vi "Assignment server.vi"() -> ()   [LabVIEW 2023]
uses:
  Control 1 server.ctl
  <vilib>/Utility/file.llb/Read Delimited Spreadsheet (string).vi
  <vilib>/Utility/file.llb/Write Delimited Spreadsheet (string).vi
  <vilib>/regexp/Match Regular Expression.xnode
panel:
  in  "Tab Control":enum32{"Page 1", "Page 2", "Page 3"}(tab)
  in  "Edit Users":bool
  in  "View Log":bool
  in  "Home Users":bool
  in  "Update users":bool
  in  "Users":string[][](table)
  out "Economy Sales":dbl
  out "Deluxe Sales":dbl
  out "Total Sales":dbl
  in  "Purchase Log":string[][](table)
  in  "Home Purchase":bool
  out "login status":dbl
  out "Logged in?":bool
  out "Password":string
  out "Username":string
  # "ADMIN DASHBOARD"
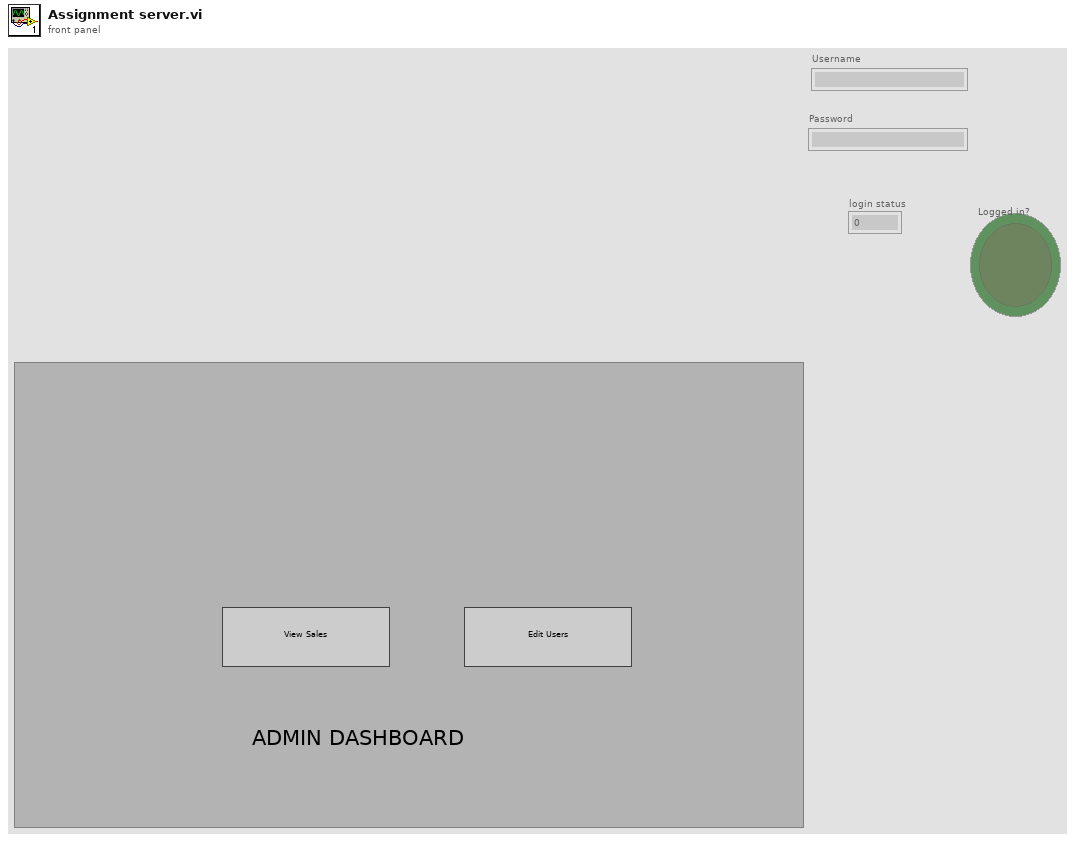
[diagram p1: front panel]
types:
  T1 = typedef "Control 1 server.ctl" = enum16{"init", "login", "logging", "pre-init"}
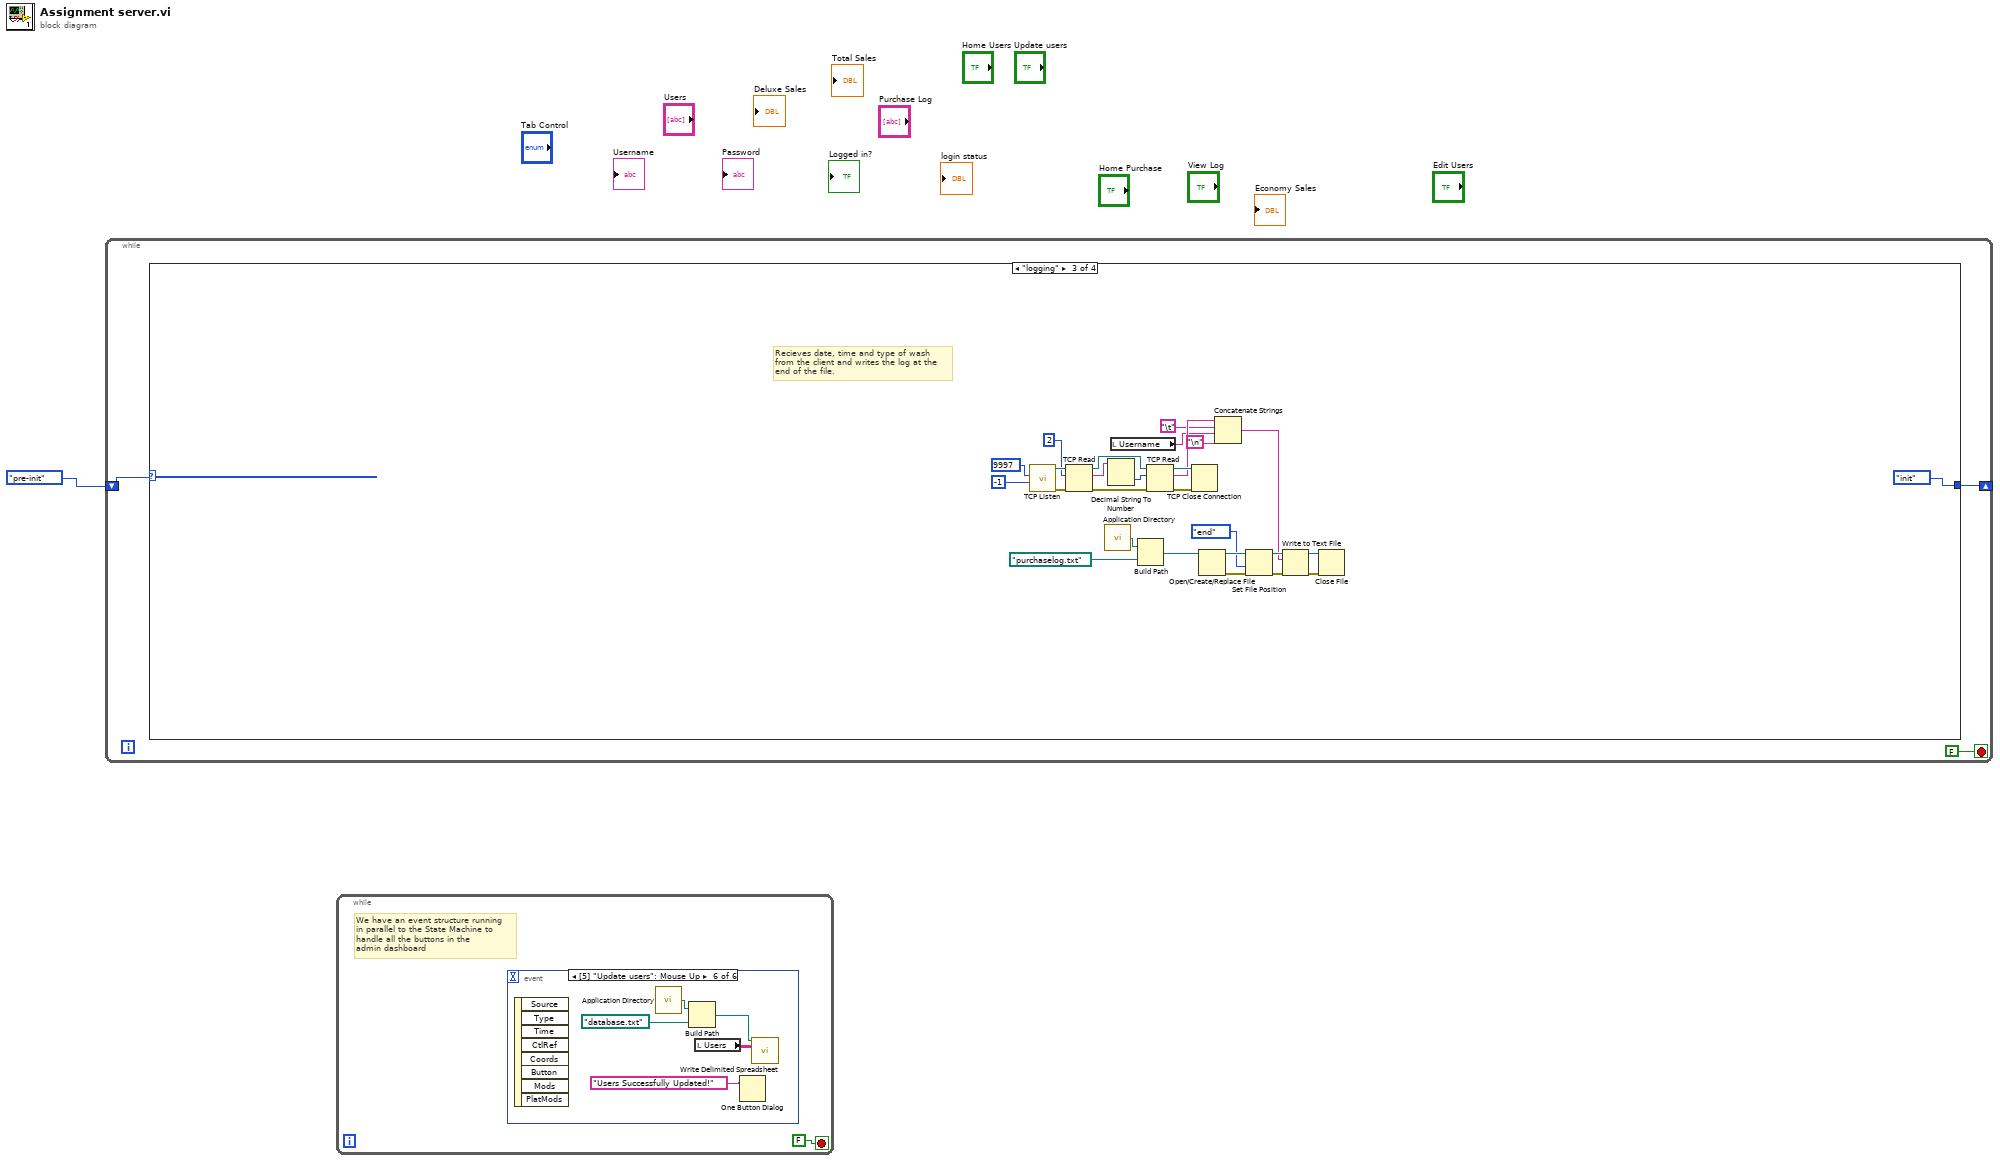
[diagram p0: block diagram]
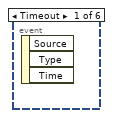
[diagram p2: hidden frame]
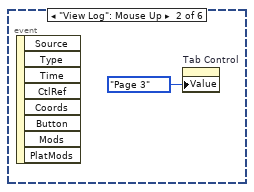
[diagram p3: hidden frame]
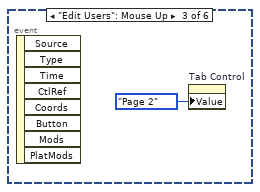
[diagram p4: hidden frame]
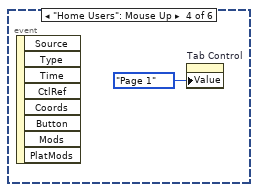
[diagram p5: hidden frame]
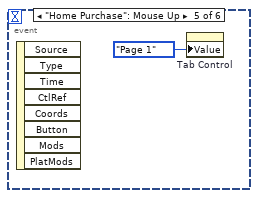
[diagram p6: hidden frame]
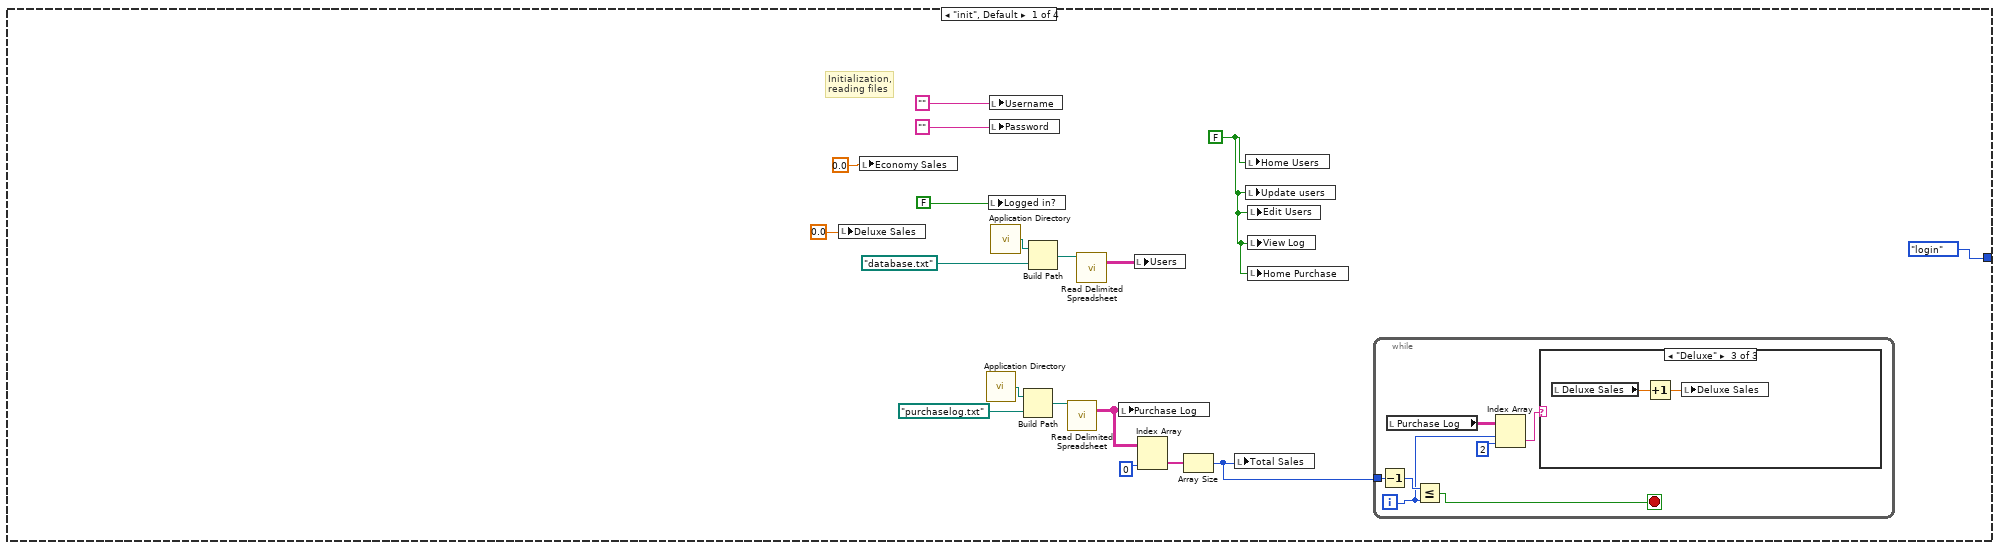
[diagram p7: hidden frame]
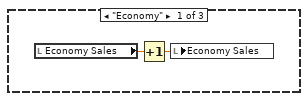
[diagram p8: hidden frame]
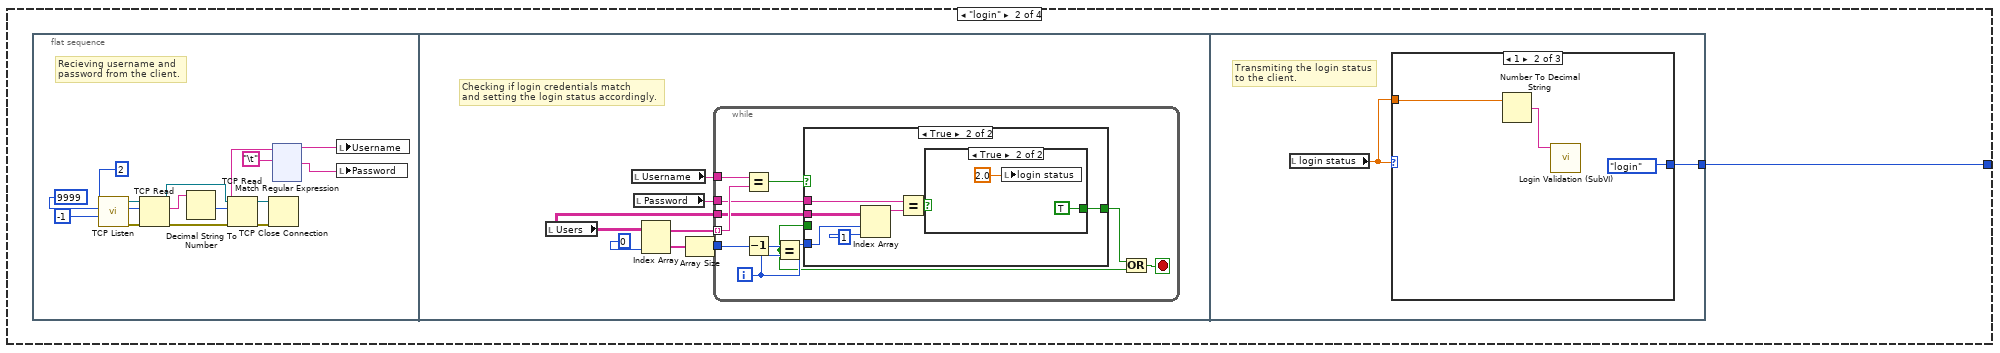
[diagram p10: hidden frame]
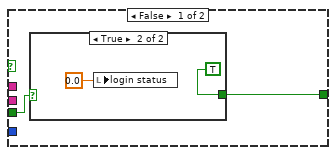
[diagram p11: hidden frame]
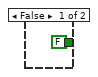
[diagram p12: hidden frame]
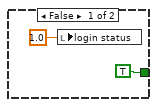
[diagram p13: hidden frame]
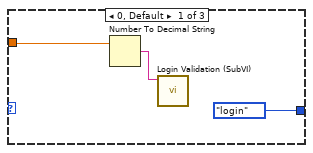
[diagram p14: hidden frame]
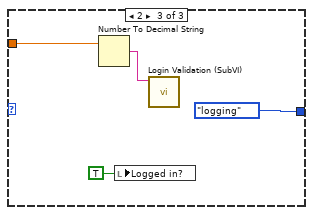
[diagram p15: hidden frame]
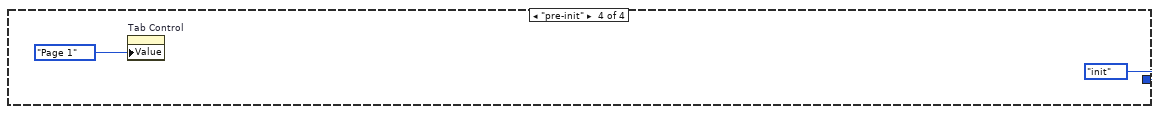
[diagram p16: hidden frame]
diagram:
  n1 = while {
    shift-right: [w2] -> _
    shift-left: Control_1_server."pre-init" -> [w3]
    stop <- FALSE stop-if-true
    n2 = case shown="\"logging\"" w3 {
      tunnel: [Control_1_server."login" w34 Control_1_server."init" Control_1_server."init"] -> w2
      frame "init", Default {
        w12 = FALSE ("Home Users")
        # "Initialization,\nreading files"
        n3 = local write "Deluxe Sales"(0.0 ("Economy Sales:")) -> ()
        n4 = local write "Economy Sales"(0.0 ("Economy Sales:")) -> ()
        n5 = call <vilib>:"Application Directory.vi"() -> ("Application Directory"=w13:path)
        n6 = local write "Logged in?"(FALSE ("Logged in?")) -> ()
        n7 = local write "Username"("" ("Username")) -> ()
        n8 = local write "Password"("" ("Password")) -> ()
        n9 = call <vilib>:"Application Directory.vi"() -> ("Application Directory"=w14:path)
        n10 = Build Path(base path=w13, name or relative path=path "purchaselog.txt") -> (appended path=w15:path)
        n11 = Build Path(base path=w14, name or relative path=path "database.txt") -> (appended path=w17:path)
        n12 = call-poly <vilib>:"Read Delimited Spreadsheet.vi"("file path (dialog if empty)"=w15) -> ("all rows"=w8:string[][])  [unwired: 9 in, 5 out]
        n13 = call-poly <vilib>:"Read Delimited Spreadsheet.vi"("file path (dialog if empty)"=w17) -> ("all rows"=w11:string[][])  [unwired: 9 in, 5 out]
        n14 = local write "Purchase Log"(w8) -> ()
        n15 = local write "Users"(w11) -> ()
        n16 = Index Array(array=w8, index (col)=0) -> (element=w10:string[])  [unwired: 1 in]
        n17 = Array Size(array=w10) -> (size(s)=w7:i32)
        n18 = local write "Total Sales"(w7) -> ()
        n19 = local write "Home Users"(w12) -> ()
        n20 = local write "Update users"(w12) -> ()
        n21 = local write "Edit Users"(w12) -> ()
        n22 = local write "View Log"(w12) -> ()
        n23 = local write "Home Purchase"(w12) -> ()
        n24 = while {
          tunnel: w7 -> [w27]
          i -> [w24]
          stop <- w23 stop-if-true
          n25 = Decrement(x=w27) -> (x-1=w25:i32)
          n26 = local read "Purchase Log"() -> (w29:string[][])
          n27 = Less Or Equal?(x=w25, y=w24) -> (x <= y?=w23:bool)
          n28 = Index Array(array=w29, index (row)=w24, index (col)=2) -> (element=w26:string)
          n29 = case shown="\"Deluxe\"" w26 {
            frame "Economy" {
              n30 = local read "Economy Sales"() -> (w31:dbl)
              n31 = Increment(x=w31) -> (x+1=w30:dbl)
              n32 = local write "Economy Sales"(w30) -> ()
            }
            frame Default {
            }
            frame "Deluxe" {
              n33 = local read "Deluxe Sales"() -> (w33:dbl)
              n34 = Increment(x=w33) -> (x+1=w32:dbl)
              n35 = local write "Deluxe Sales"(w32) -> ()
            }
          }
        }
      }
      frame "login" {
        n36 = flat-sequence {
          tunnel: [w200] -> w34
          frame #0 {
            # "Recieving username and\npassword from the client."
            n37 = call <vilib>:"TCP Listen.vi"("timeout ms (wait forever: -1)"=-1, "port"=u16 9999) -> ("error out"=w48:errorcluster, "connection ID"=w49:refnum<k5>)  [unwired: 5 in, 3 out]
            n38 = TCP Read(connection ID=w49, bytes to read=2, error in (no error)=w48) -> (connection ID out=w36:refnum<k5>, data out=w35:string, error out=w47:errorcluster)  [unwired: 2 in]
            n39 = Decimal String To Number(string=w35) -> (number=w44:i32)  [unwired: 2 in, 1 out]
            n40 = TCP Read(connection ID=w36, bytes to read=w44, error in (no error)=w47) -> (connection ID out=w45:refnum<k5>, data out=w43:string, error out=w46:errorcluster)  [unwired: 2 in]
            n41 = TCP Close Connection(connection ID=w45, error in (no error)=w46) -> ()  [unwired: 1 in, 2 out]
            n42 = xnode ("Match Regular Expression")("input string"=w43, "regular expression"="\t") -> ("before match"=w38:string, "after match"=w37:string)  [unwired: 4 in, 3 out]
            n43 = local write "Username"(w38) -> ()
            n44 = local write "Password"(w37) -> ()
          }
          frame #1 {
            # "Checking if login credentials match\nand setting the login status accordingly."
            n45 = local read "Users"() -> (w170:string[][])
            n46 = local read "Username"() -> (w168:string)
            n47 = local read "Password"() -> (w167:string)
            n48 = Index Array(array=w170, index (col)=0 ("index (row)")) -> (element=w171:string[])  [unwired: 1 in]
            n49 = Array Size(array=w171) -> (size(s)=w172:i32)
            n50 = while {
              tunnel: w172 -> [w183]
              tunnel: w171 -> [w181] mode=indexing
              tunnel: w170 -> [w179]
              tunnel: w168 -> [w174]
              tunnel: w167 -> [w173]
              i -> [w178]
              stop <- w177 stop-if-true
              n51 = Equal?(x=w174, y=w181) -> (x = y?=w180:bool)
              n52 = Decrement(x=w183) -> (x-1=w182:i32)
              n53 = Equal?(x=w182, y=w178) -> (x = y?=w175:bool)
              n54 = case shown="True" w180 {
                tunnel: w179 -> [_ w195]
                tunnel: w178 -> [_ w192]
                tunnel: [w184 w190] -> w176
                tunnel: w175 -> [w185 _]
                tunnel: w173 -> [_ w189]
                frame False {
                  n55 = case shown="True" w185 {
                    tunnel: [FALSE TRUE] -> w184
                    frame False {
                    }
                    frame True {
                      n56 = local write "login status"(0.0 ("login status")) -> ()
                    }
                  }
                }
                frame True {
                  n57 = Index Array(array=w195, index (row)=w192, index (col)=1) -> (element=w193:string)
                  n58 = Equal?(x=w189, y=w193) -> (x = y?=w191:bool)
                  n59 = case shown="True" w191 {
                    tunnel: [TRUE TRUE ("Logged in?")] -> w190
                    frame False {
                      n60 = local write "login status"(1.0 ("login status")) -> ()
                    }
                    frame True {
                      n61 = local write "login status"(2.0 ("login status")) -> ()
                    }
                  }
                }
              }
              n62 = Or(x=w176, y=w175) -> (x .or. y?=w177:bool)
            }
          }
          frame #2 {
            # "Transmiting the login status\nto the client."
            n63 = local read "login status"() -> (w201:dbl)
            n64 = case shown="1" w201 {
              tunnel: [Control_1_server."login" Control_1_server."login" Control_1_server."logging"] -> w200
              tunnel: w201 -> [w203 w206 w210]
              frame 0, Default {
                n65 = Number To Decimal String(number=w203) -> (decimal integer string=w202:string)  [unwired: 1 in]
                n66 = call "Login Validation (SubVI).vi"("String"=w202) -> ()  [unwired: 11 in]
              }
              frame 1 {
                n67 = Number To Decimal String(number=w206) -> (decimal integer string=w205:string)  [unwired: 1 in]
                n68 = call "Login Validation (SubVI).vi"("String"=w205) -> ()  [unwired: 11 in]
              }
              frame 2 {
                n69 = Number To Decimal String(number=w210) -> (decimal integer string=w208:string)  [unwired: 1 in]
                n70 = local write "Logged in?"(TRUE ("Logged in?")) -> ()
                n71 = call "Login Validation (SubVI).vi"("String"=w208) -> ()  [unwired: 11 in]
              }
            }
          }
        }
      }
      frame "logging" {
        # "Recieves date, time and type of wash\nfrom the client and writes the log at the\nend of the file."
        n72 = call <vilib>:"TCP Listen.vi"("timeout ms (wait forever: -1)"=-1, "port"=u16 9997) -> ("error out"=w235:errorcluster, "connection ID"=w238:refnum<k5>)  [unwired: 5 in, 3 out]
        n73 = TCP Read(connection ID=w238, bytes to read=2, error in (no error)=w235) -> (connection ID out=w237:refnum<k5>, data out=w231:string, error out=w234:errorcluster)  [unwired: 2 in]
        n74 = call <vilib>:"Application Directory.vi"() -> ("Application Directory"=w221:path)
        n75 = Decimal String To Number(string=w231) -> (number=w232:i32)  [unwired: 2 in, 1 out]
        n76 = local read "Username"() -> (w223:string)
        n77 = Build Path(base path=w221, name or relative path=path "purchaselog.txt") -> (appended path=w220:path)
        n78 = TCP Read(connection ID=w237, bytes to read=w232, error in (no error)=w234) -> (connection ID out=w236:refnum<k5>, data out=w224:string, error out=w233:errorcluster)  [unwired: 2 in]
        n79 = TCP Close Connection(connection ID=w236, error in (no error)=w233) -> ()  [unwired: 1 in, 2 out]
        n80 = Open/Create/Replace File(file path (use dialog)=w220) -> (refnum out=w230:refnum<file>, error out=w229:errorcluster)  [unwired: 5 in, 1 out]
        n81 = Concatenate Strings(w224, "\t", w223, "\n") -> (w222:string)
        n82 = Set File Position(refnum=w230, from (0:start)=enum16{"start", "end", "current"}."end", error in=w229) -> (refnum out=w228:refnum<file>, error out=w227:errorcluster)  [unwired: 1 in]
        n83 = Write to Text File(file (use dialog)=w228, text=w222, error in=w227) -> (refnum out=w225:refnum<file>, error out=w226:errorcluster)  [unwired: 1 in, 1 out]
        n84 = Close File(refnum=w225, error in=w226) -> ()  [unwired: 2 out]
      }
      frame "pre-init" {
        n85 = property on="Tab Control" class="TabCtl (strict)"("Value"=enum32{"Page 1", "Page 2", "Page 3"}."Page 1" ("Tab Control")) -> ()  [unwired: 2 in, 2 out]
      }
    }
  }
  n86 = while {
    stop <- FALSE stop-if-true
    # "We have an event structure running \nin parallel to the State Machine to\nhandle all the buttons in the \nadmin dashboard"
    n87 = event shown="[5] \"Update users\": Mouse Up" {
      selector: _ -> [_ _ _ _ _ _]
      dyn-events: _ -> [_ _ _ _ _ _]
      timeout: _ -> [_ _ _ _ _ _]
      event Timeout {
        n88 = event-data() -> ()  [unwired: 1 in, 3 out]
      }
      event "View Log": Mouse Up {
        n89 = event-data() -> ()  [unwired: 1 in, 8 out]
        n90 = property on="Tab Control" class="TabCtl (strict)"("Value"=enum32{"Page 1", "Page 2", "Page 3"}."Page 3" ("Tab Control")) -> ()  [unwired: 2 in, 2 out]
      }
      event "Edit Users": Mouse Up {
        n91 = event-data() -> ()  [unwired: 1 in, 8 out]
        n92 = property on="Tab Control" class="TabCtl (strict)"("Value"=enum32{"Page 1", "Page 2", "Page 3"}."Page 2" ("Tab Control")) -> ()  [unwired: 2 in, 2 out]
      }
      event "Home Users": Mouse Up {
        n93 = event-data() -> ()  [unwired: 1 in, 8 out]
        n94 = property on="Tab Control" class="TabCtl (strict)"("Value"=enum32{"Page 1", "Page 2", "Page 3"}."Page 1" ("Tab Control")) -> ()  [unwired: 2 in, 2 out]
      }
      event "Home Purchase": Mouse Up {
        n95 = event-data() -> ()  [unwired: 1 in, 8 out]
        n96 = property on="Tab Control" class="TabCtl (strict)"("Value"=enum32{"Page 1", "Page 2", "Page 3"}."Page 1" ("Tab Control")) -> ()  [unwired: 2 in, 2 out]
      }
      event "Update users": Mouse Up {
        n97 = event-data() -> ()  [unwired: 1 in, 8 out]
        n98 = call <vilib>:"Application Directory.vi"() -> ("Application Directory"=w248:path)
        n99 = Build Path(base path=w248, name or relative path=path "database.txt") -> (appended path=w249:path)
        n100 = local read "Users"() -> (w247:string[][])
        n101 = One Button Dialog(message="Users Successfully Updated!") -> ()  [unwired: 1 in, 1 out]
        n102 = call-poly <vilib>:"Write Delimited Spreadsheet.vi"("file path (dialog if empty)"=w249, "2D data"=w247) -> ()  [unwired: 12 in, 2 out]
      }
    }
  }
